vi "FM Demod RTLSDR DLL.vi"(8 "error in (no error)":errorcluster, 9 "Baseband":dbl[](array[numeric])=array[35829 elements], 10 "QSamples":dbl[](array[numeric])=array[35830 elements], 11 "ISamples":dbl[](array[numeric])=array[35830 elements]) -> (0 "error out":errorcluster, 1 "Baseband out":dbl[](array[numeric]))   [LabVIEW 2013, in "FMDemodRTLSDR_DLL.lvlib"]
doc: "extern void FMDemodRTLSDR_DLL(const double ISamples[35830], const double\n QSamples[35830], double Baseband[35829]);"
uses:
  <userlib>/FMDemodRTLSDR_DLL/FMDemodRTLSDR_DLL.lvlib
  <userlib>/FMDemodRTLSDR_DLL/FMDemodRTLSDR_DLL.dll
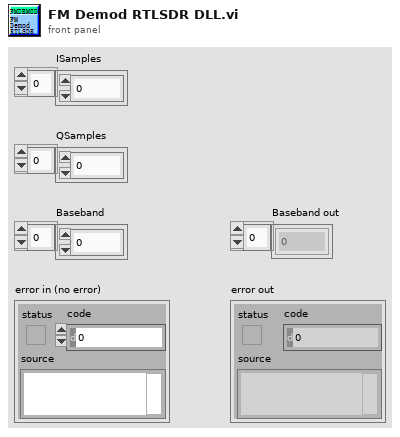
[diagram p1: front panel]
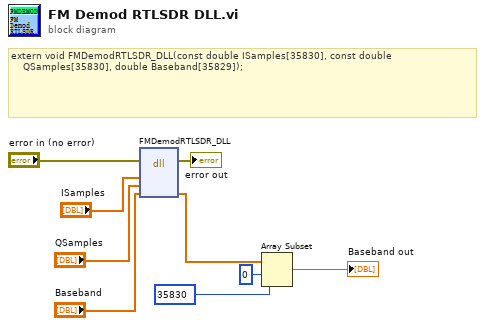
[diagram p0: block diagram]
diagram:
  # "extern void FMDemodRTLSDR_DLL(const double ISamples[35830], const double\n    QSamples[35830], double Baseband[35829]);"
  n1 = dll-call lib="C:/Program Files/National Instruments/LabVIEW 2013/user.lib/FMDemodRTLSDR_DLL/FMDemodRTLSDR_DLL.*" fn="FMDemodRTLSDR_DLL"(error in="error in (no error)", "ISamples"="ISamples", "QSamples"="QSamples", "Baseband"="Baseband") -> (error out=→"error out":errorcluster, "Baseband"=w4:dbl[])  [unwired: 5 in, 1 out]
  n2 = Array Subset(array=w4, index=0, length=35830) -> (→"Baseband out":dbl[])
